vi "Tx Disable channel logic 4ch.vi"(5 "num channels":u32, 6 "ready for output":bool, 9 "input valid":bool, 10 "data in":u32[](array[numeric])=[0, 0, 0, 0], 11 "enabled channels":u32) -> (0 "enable new data":bool, 1 "output valid":bool, 2 "data out":u32[](array[numeric]))   [LabVIEW 2025, in "niUSRP Stream Control (DMA) v1 FPGA.lvclass"]
uses:
  niUSRP Stream Control (DMA) v1 FPGA.lvclass
  niUSRP Stream Control (DMA) v1 FPGA.lvclass/niUSRP Stream Control (DMA) v1 FPGA.ctl
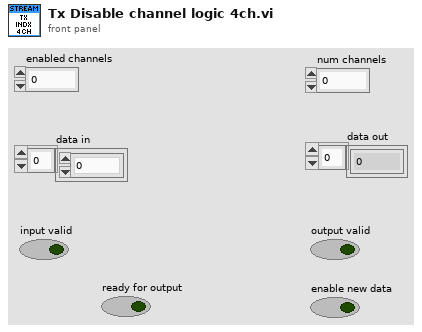
[diagram p1: front panel]
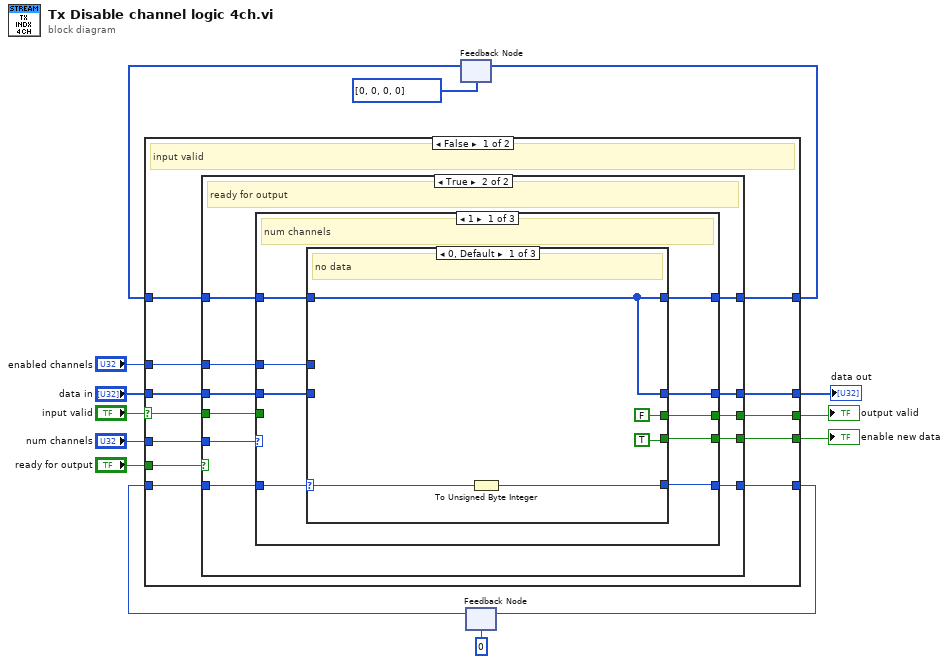
[diagram p0: block diagram]
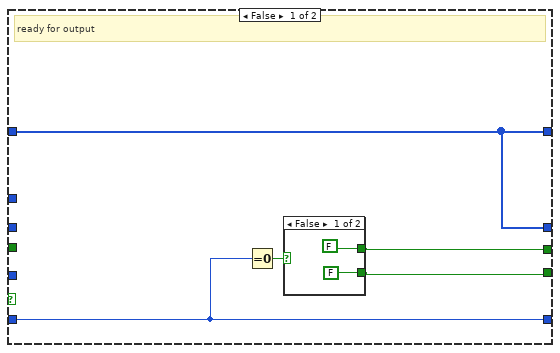
[diagram p2: hidden frame]
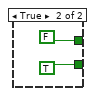
[diagram p3: hidden frame]
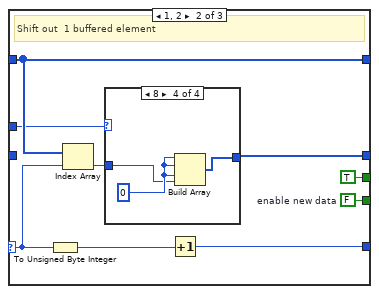
[diagram p4: hidden frame]
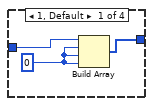
[diagram p5: hidden frame]
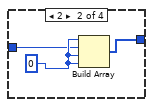
[diagram p6: hidden frame]
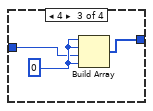
[diagram p7: hidden frame]
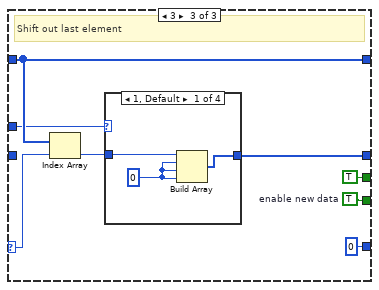
[diagram p8: hidden frame]
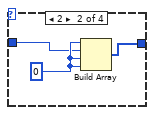
[diagram p9: hidden frame]
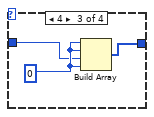
[diagram p10: hidden frame]
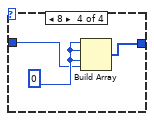
[diagram p11: hidden frame]
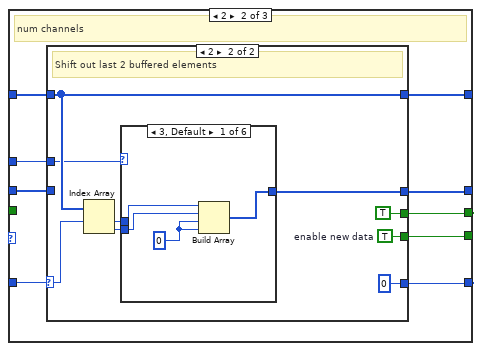
[diagram p12: hidden frame]
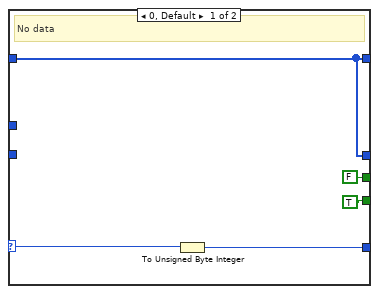
[diagram p13: hidden frame]
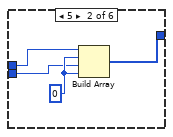
[diagram p14: hidden frame]
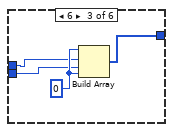
[diagram p15: hidden frame]
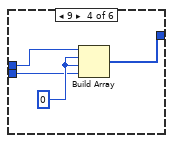
[diagram p16: hidden frame]
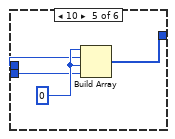
[diagram p17: hidden frame]
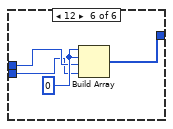
[diagram p18: hidden frame]
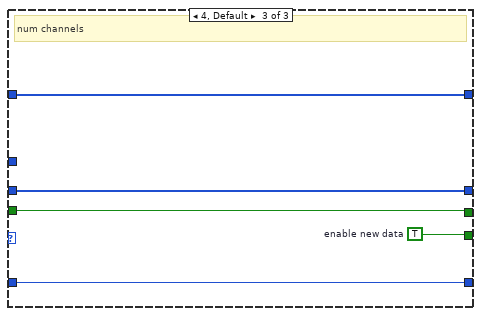
[diagram p19: hidden frame]
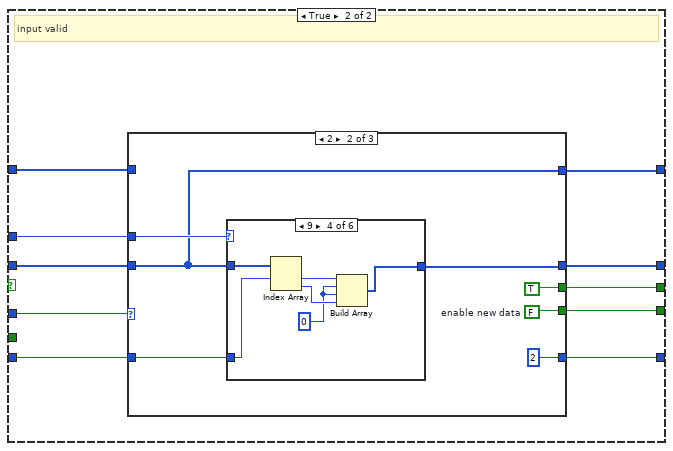
[diagram p20: hidden frame]
diagram:
  n1 = feedback #1(u32[] [0, 0, 0, 0]) -> (w12:u32[])
  n2 = feedback #2(u8 0) -> (w2:u8)
  n3 = case shown="False" "input valid" {
    selector: "input valid" -> [w16 _]
    tunnel: "num channels" -> [w26 w163]
    tunnel: [w25 w159] -> w9
    tunnel: [w24 w158] -> w8
    tunnel: "data in" -> [w23 w160]
    tunnel: "enabled channels" -> [w22 w155]
    tunnel: [w21 w157] -> w10
    tunnel: w12 -> [w20 w154]
    tunnel: [w19 w156] -> w11
    tunnel: [w17 w162] -> w1
    tunnel: w2 -> [w18 w161]
    tunnel: "ready for output" -> [w15 _]
    frame False {
      # "input valid"
      n4 = case shown="True" w15 {
        tunnel: w26 -> [_ w46]
        tunnel: [w30 w45] -> w25
        tunnel: [w29 w44] -> w24
        tunnel: w23 -> [_ w43]
        tunnel: w22 -> [_ w42]
        tunnel: [w28 w41] -> w21
        tunnel: w20 -> [w28 w40]
        tunnel: [w28 w39] -> w19
        tunnel: w18 -> [w27 w38]
        tunnel: [w27 w37] -> w17
        tunnel: w16 -> [_ w36]
        frame False {
          # "ready for output"
          n5 = Equal To 0?(x=w27) -> (x = 0?=w31:bool)
          n6 = case shown="False" w31 {
            tunnel: [FALSE TRUE] -> w29
            tunnel: [FALSE FALSE] -> w30
            frame False {
            }
            frame True {
            }
          }
        }
        frame True {
          # "ready for output"
          n7 = case shown="1" w46 {
            tunnel: w42 -> [w55 w109 _]
            tunnel: w43 -> [w54 w110 w153]
            tunnel: [w53 w106 w152] -> w44
            tunnel: [w52 w107 w149] -> w45
            tunnel: [w51 w108 w153] -> w41
            tunnel: w40 -> [w47 w102 w150]
            tunnel: [w50 w103 w150] -> w39
            tunnel: w38 -> [w49 w104 w151]
            tunnel: [w48 w105 w151] -> w37
            tunnel: w36 -> [_ _ w149]
            frame 1 {
              # "num channels"
              n8 = case shown="0, Default" w49 {
                selector: w49 -> [w59 w66 w85]
                tunnel: w54 -> [_ _ _]
                tunnel: [w56 w69 u8 0] -> w48
                tunnel: [w57 w68 w84] -> w51
                tunnel: [FALSE TRUE TRUE] -> w52
                tunnel: w47 -> [w57 w65 w86]
                tunnel: [w57 w65 w86] -> w50
                tunnel: [TRUE w64 w87] -> w53
                tunnel: w55 -> [_ w63 w83]
                frame 0, Default {
                  # "no data"
                  n9 = To Unsigned Byte Integer(number=w59) -> (unsigned 8bit integer=w56:u8)
                }
                frame 1, 2 {
                  w64 = FALSE  # enable new data
                  # "Shift out  1 buffered element"
                  n10 = To Unsigned Byte Integer(number=w66) -> (unsigned 8bit integer=w61:u8)
                  n11 = Index Array(array=w65, index=w66) -> (element=w62:u32)
                  n12 = case shown="8" w63 {
                    tunnel: [w72 w75 w78 w81] -> w68
                    tunnel: w62 -> [w70 w73 w76 w79]
                    frame 1, Default {
                      w71 = u32 0
                      n13 = Build Array(w70, w71, w71, w71) -> (w72:u32[])
                    }
                    frame 2 {
                      w74 = u32 0
                      n14 = Build Array(w74, w73, w74, w74) -> (w75:u32[])
                    }
                    frame 4 {
                      w77 = u32 0
                      n15 = Build Array(w77, w77, w76, w77) -> (w78:u32[])
                    }
                    frame 8 {
                      w80 = u32 0
                      n16 = Build Array(w80, w80, w80, w79) -> (w81:u32[])
                    }
                  }
                  n17 = Increment(x=w61) -> (x+1=w69:u8)
                }
                frame 3 {
                  w87 = TRUE  # enable new data
                  # "Shift out last element"
                  n18 = Index Array(array=w86, index=w85) -> (element=w82:u32)
                  n19 = case shown="1, Default" w83 {
                    tunnel: [w92 w95 w98 w101] -> w84
                    tunnel: w82 -> [w90 w93 w96 w99]
                    frame 1, Default {
                      w91 = u32 0
                      n20 = Build Array(w90, w91, w91, w91) -> (w92:u32[])
                    }
                    frame 2 {
                      w94 = u32 0
                      n21 = Build Array(w94, w93, w94, w94) -> (w95:u32[])
                    }
                    frame 4 {
                      w97 = u32 0
                      n22 = Build Array(w97, w97, w96, w97) -> (w98:u32[])
                    }
                    frame 8 {
                      w100 = u32 0
                      n23 = Build Array(w100, w100, w100, w99) -> (w101:u32[])
                    }
                  }
                }
              }
            }
            frame 2 {
              # "num channels"
              n24 = case shown="2" w104 {
                selector: w104 -> [w114 w120]
                tunnel: w110 -> [_ _]
                tunnel: [w113 u8 0] -> w105
                tunnel: [w111 w118] -> w108
                tunnel: [FALSE TRUE] -> w107
                tunnel: w102 -> [w111 w121]
                tunnel: [w111 w121] -> w103
                tunnel: [TRUE w122] -> w106
                tunnel: w109 -> [_ w119]
                frame 0, Default {
                  # "No data"
                  n25 = To Unsigned Byte Integer(number=w114) -> (unsigned 8bit integer=w113:u8)
                }
                frame 2 {
                  w122 = TRUE  # enable new data
                  # "Shift out last 2 buffered elements"
                  n26 = Index Array(array=w121, index #1=w120) -> (element #1=w117:u32, element #2=w116:u32)  [unwired: 1 in]
                  n27 = case shown="3, Default" w119 {
                    tunnel: [w128 w132 w136 w140 w144 w148] -> w118
                    tunnel: w117 -> [w126 w130 w134 w138 w142 w146]
                    tunnel: w116 -> [w125 w129 w133 w137 w141 w145]
                    frame 3, Default {
                      w127 = u32 0
                      n28 = Build Array(w126, w125, w127, w127) -> (w128:u32[])
                    }
                    frame 5 {
                      w131 = u32 0
                      n29 = Build Array(w130, w131, w129, w131) -> (w132:u32[])
                    }
                    frame 6 {
                      w135 = u32 0
                      n30 = Build Array(w135, w134, w133, w135) -> (w136:u32[])
                    }
                    frame 9 {
                      w139 = u32 0
                      n31 = Build Array(w138, w139, w139, w137) -> (w140:u32[])
                    }
                    frame 10 {
                      w143 = u32 0
                      n32 = Build Array(w143, w142, w143, w141) -> (w144:u32[])
                    }
                    frame 12 {
                      w147 = u32 0
                      n33 = Build Array(w147, w147, w146, w145) -> (w148:u32[])
                    }
                  }
                }
              }
            }
            frame 4, Default {
              w152 = TRUE  # enable new data
              # "num channels"
            }
          }
        }
      }
    }
    frame True {
      # "input valid"
      n34 = case shown="2" w163 {
        tunnel: [w169 i8 2 ("length") i8 0 ("length")] -> w162
        tunnel: w161 -> [_ w191 _]
        tunnel: w160 -> [w165 w192 w235]
        tunnel: [TRUE TRUE TRUE] -> w159
        tunnel: [w167 w194 w237] -> w158
        tunnel: [w166 w196 w235] -> w157
        tunnel: [w165 w192 w234] -> w156
        tunnel: w155 -> [w164 w197 _]
        tunnel: w154 -> [_ _ w234]
        frame 1, Default {
          w167 = FALSE  # enable new data
          w170 = i8 0
          n35 = case shown="1, Default" w164 {
            tunnel: [w172 w178 w183 w188] -> w166
            tunnel: w170 -> [w175 w180 w185 w190]
            tunnel: w165 -> [w174 w179 w184 w189]
            frame 1, Default {
              w171 = u32 0
              n36 = Index Array(array=w174, index=w175) -> (element=w173:u32)
              n37 = Build Array(w173, w171, w171, w171) -> (w172:u32[])
            }
            frame 2 {
              w176 = u32 0
              n38 = Index Array(array=w179, index=w180) -> (element=w177:u32)
              n39 = Build Array(w176, w177, w176, w176) -> (w178:u32[])
            }
            frame 4 {
              w181 = u32 0
              n40 = Index Array(array=w184, index=w185) -> (element=w182:u32)
              n41 = Build Array(w181, w181, w182, w181) -> (w183:u32[])
            }
            frame 8 {
              w186 = u32 0
              n42 = Index Array(array=w189, index=w190) -> (element=w187:u32)
              n43 = Build Array(w186, w186, w186, w187) -> (w188:u32[])
            }
          }
          n44 = Increment(x=w170) -> (x+1=w169:i8)
        }
        frame 2 {
          w194 = FALSE  # enable new data
          n45 = case shown="9" w197 {
            tunnel: w192 -> [w203 w208 w215 w221 w227 w233]
            tunnel: [w202 w207 w214 w220 w226 w232] -> w196
            tunnel: w191 -> [w199 w206 w213 w217 w225 w229]
            frame 3, Default {
              w198 = u32 0
              n46 = Index Array(array=w203, index #1=w199) -> (element #1=w201:u32, element #2=w200:u32)  [unwired: 1 in]
              n47 = Build Array(w201, w200, w198, w198) -> (w202:u32[])
            }
            frame 5 {
              w204 = u32 0
              n48 = Index Array(array=w208, index #1=w206) -> (element #1=w209:u32, element #2=w205:u32)  [unwired: 1 in]
              n49 = Build Array(w209, w204, w205, w204) -> (w207:u32[])
            }
            frame 6 {
              w210 = u32 0
              n50 = Index Array(array=w215, index #1=w213) -> (element #1=w212:u32, element #2=w211:u32)  [unwired: 1 in]
              n51 = Build Array(w210, w212, w211, w210) -> (w214:u32[])
            }
            frame 9 {
              w216 = u32 0
              n52 = Index Array(array=w221, index #1=w217) -> (element #1=w219:u32, element #2=w218:u32)  [unwired: 1 in]
              n53 = Build Array(w219, w216, w216, w218) -> (w220:u32[])
            }
            frame 10 {
              w222 = u32 0
              n54 = Index Array(array=w227, index #1=w225) -> (element #1=w224:u32, element #2=w223:u32)  [unwired: 1 in]
              n55 = Build Array(w222, w224, w222, w223) -> (w226:u32[])
            }
            frame 12 {
              w228 = u32 0
              n56 = Index Array(array=w233, index #1=w229) -> (element #1=w231:u32, element #2=w230:u32)  [unwired: 1 in]
              n57 = Build Array(w228, w228, w231, w230) -> (w232:u32[])
            }
          }
        }
        frame 4 {
          w237 = TRUE  # enable new data
        }
      }
    }
  }
  "output valid" <- w9
  "enable new data" <- w8
  "data out" <- w10
  n58 = feedback-in #1(w11) -> ()
  n59 = feedback-in #2(w1) -> ()
